vi "Chain of Responsiblility Example.vi"() -> ()   [LabVIEW 2014]
uses:
  user.lib/_NEVSTOP/Communicable State Machine(CSM)/_Support/Typedef/_CSM_MODE.ctl
  user.lib/_NEVSTOP/Communicable State Machine(CSM)/_Support/Priority Queue/Priority Queue.lvclass/Priority Queue.ctl
  user.lib/_NEVSTOP/Communicable State Machine(CSM)/_Support/Typedef/_CSM_GlobalLog_MSG.ctl
  user.lib/_NEVSTOP/Communicable State Machine(CSM)/_Support/Typedef/_CSM_Response Source Message.ctl
  user.lib/_NEVSTOP/Communicable State Machine(CSM)/_Support/Typedef/_CSM_GlobalLog_MSG_TYPE.ctl
  user.lib/_NEVSTOP/Communicable State Machine(CSM)/_Support/CSMQ/_Obtain CSM Data Queue.vi
  user.lib/_NEVSTOP/Communicable State Machine(CSM)/_Support/Priority Queue/Release Priority Queue.vi
  user.lib/_NEVSTOP/Communicable State Machine(CSM)/_Support/Priority Queue/Not a Refnum.vi
  user.lib/_NEVSTOP/Communicable State Machine(CSM)/_Support/Process/CSMP-Async Call.vi
  user.lib/_NEVSTOP/Communicable State Machine(CSM)/_Support/GlobalEvent/GEvt-Generate Status Log.vi
  user.lib/_NEVSTOP/Communicable State Machine(CSM)/_Support/Process/CSMP-Broadcast.vi
  user.lib/_NEVSTOP/Communicable State Machine(CSM)/_Support/GlobalEvent/GEvt-Generate Interrupt Log.vi
  user.lib/_NEVSTOP/Communicable State Machine(CSM)/_Support/GlobalEvent/GEvt-Generate Register Log.vi
  user.lib/_NEVSTOP/Communicable State Machine(CSM)/_Support/Process/CSMP-Register Status.vi
  user.lib/_NEVSTOP/Communicable State Machine(CSM)/_Support/GlobalEvent/GEvt-Generate Unregister Log.vi
  user.lib/_NEVSTOP/Communicable State Machine(CSM)/_Support/Process/CSMP-Unregister Status.vi
  user.lib/_NEVSTOP/Communicable State Machine(CSM)/_Support/Process/CSMP-Sync Call.vi
  user.lib/_NEVSTOP/Communicable State Machine(CSM)/_Support/CSMQ/_CSMObj-Unlock.vi
  user.lib/_NEVSTOP/Communicable State Machine(CSM)/_Support/Process/CSMP-PostPostMsg.vi
  user.lib/_NEVSTOP/Communicable State Machine(CSM)/_Support/Process/CSMP-PostSendMsg.vi
  user.lib/_NEVSTOP/Communicable State Machine(CSM)/_Support/CSMQ/_CSMObj-Lock State.vi
  user.lib/_NEVSTOP/Communicable State Machine(CSM)/_Support/Common/Splite Reason String Part.vi
  user.lib/_NEVSTOP/Communicable State Machine(CSM)/_Support/Common/Trim Single line Text.vi
  user.lib/_NEVSTOP/Communicable State Machine(CSM)/_Support/CSMQ/_CSMOFGV Release.vi
  user.lib/_NEVSTOP/Communicable State Machine(CSM)/_Support/Common/Remove Comments from Line.vi
  user.lib/_NEVSTOP/Communicable State Machine(CSM)/_Support/Common/Splite Single-line Message.vi
  user.lib/_NEVSTOP/Communicable State Machine(CSM)/_Support/Common/Parse Next Single-line State.vi
  user.lib/_NEVSTOP/Communicable State Machine(CSM)/_Support/CSMQ/_CSMObj-Log Error if in a Remote Session.vi
  user.lib/_NEVSTOP/Communicable State Machine(CSM)/_Support/CSMQ/_CSMOFGV Obtain.vi
  user.lib/_NEVSTOP/Communicable State Machine(CSM)/_Support/GlobalEvent/GEvt-Generate State Change Log.vi
  user.lib/_NEVSTOP/Communicable State Machine(CSM)/_Support/GlobalEvent/GEvt-Generate Remaining States Log.vi
  user.lib/_NEVSTOP/Communicable State Machine(CSM)/_Support/GlobalEvent/GEvt-Generate Complete Log.vi
  user.lib/_NEVSTOP/Communicable State Machine(CSM)/AdvanceAPI/CSM - Revert Arguments-Safe String.vi
  user.lib/_NEVSTOP/Communicable State Machine(CSM)/_Support/Priority Queue/Obtain Priority Queue.vi
  user.lib/_NEVSTOP/Communicable State Machine(CSM)/_Support/CSMQ/_CSMObj-Message Check.vi
  user.lib/_NEVSTOP/Communicable State Machine(CSM)/_Support/FGV-BroadcastRegistry/Cache-Broadcast Registry Search Result.vi
  user.lib/_NEVSTOP/Communicable State Machine(CSM)/AdvanceAPI/CSM - Register Status Change.vi
  user.lib/_NEVSTOP/Communicable State Machine(CSM)/AdvanceAPI/CSM - Unregister Status Change.vi
  user.lib/_NEVSTOP/Communicable State Machine(CSM)/Utility/uuid.vi
  user.lib/_NEVSTOP/Communicable State Machine(CSM)/_Support/Common/CSM-Name to CSM-Mode.vi
  user.lib/_NEVSTOP/Communicable State Machine(CSM)/AdvanceAPI/CSM - Keywords.vi
  user.lib/_NEVSTOP/Communicable State Machine(CSM)/_Support/GlobalEvent/FGV-GlobalEventRef.vi
  user.lib/_NEVSTOP/Communicable State Machine(CSM)/_Support/CSMQ/_CSMOFGV.vi
  user.lib/_NEVSTOP/Communicable State Machine(CSM)/_Support/CSMQ/_CSMOFGV Dequeue.vi
  user.lib/_NEVSTOP/Communicable State Machine(CSM)/Utility/Build Error Cluster.vi
  user.lib/_NEVSTOP/Communicable State Machine(CSM)/_Support/CSMQ/_CSMObj-Enqueue Cross-Module Message.vi
  user.lib/_NEVSTOP/Communicable State Machine(CSM)/_Support/GlobalEvent/FGV-StatusChangeEventRef.vi
  user.lib/_NEVSTOP/Communicable State Machine(CSM)/_Support/FGV-BroadcastRegistry/global-Broadcast Cache Change Flag.vi
  user.lib/_NEVSTOP/Communicable State Machine(CSM)/_Support/FGV-BroadcastRegistry/FGV-BroadcastRegistry.vi
  user.lib/_NEVSTOP/Communicable State Machine(CSM)/_Support/Priority Queue/Priority Queue.lvclass
  user.lib/_NEVSTOP/Communicable State Machine(CSM)/Communicable State Machine.lvlib
panel:
  out "Array":T2(array[cluster])
  out "State History 2":string
  out "State History":string
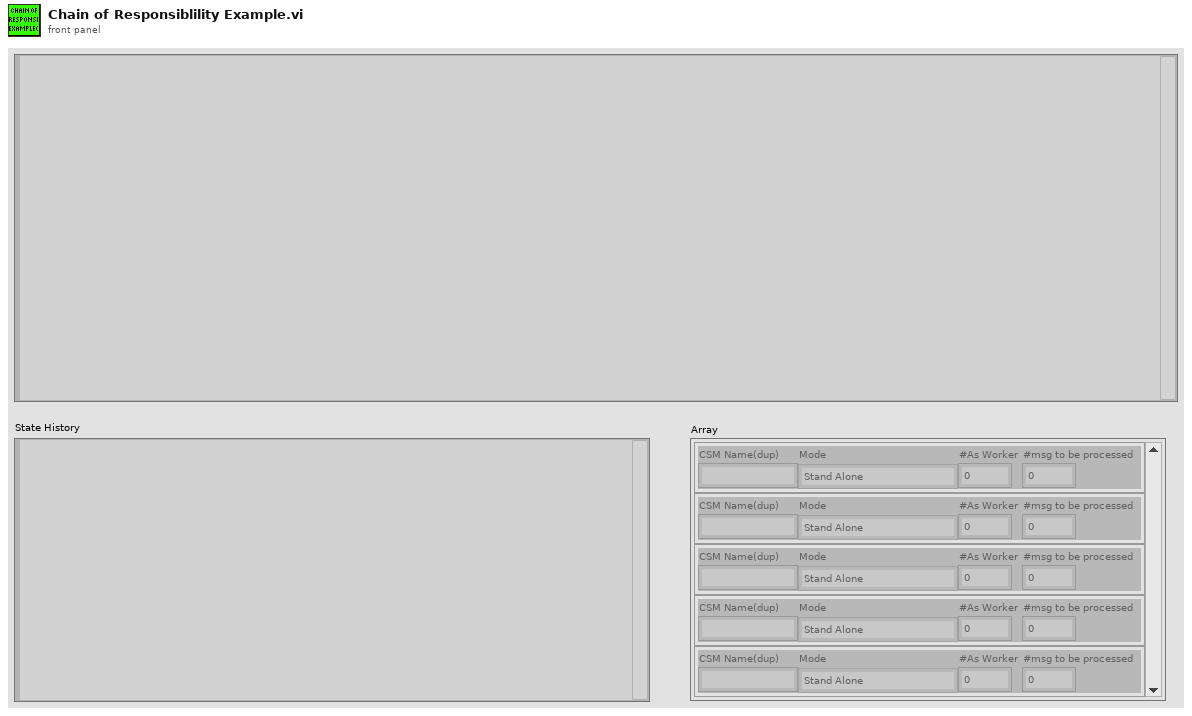
[diagram p1: front panel]
types:
  T1 = typedef "Communicable State Machine.lvlib/_CSM_MODE.ctl" = enum16{"Stand Alone", "CSM", "Action Worker", "Responsibility Chain", "Responsibility Chain Node"}
  T2 = cluster{"CSM Name(dup)":string, "Mode":T1, "#As Worker":i32, "#msg to be processed":i32}[]
  T3 = enum32{"Invalid", "Standard", "Closed", "Hidden", "Minimized", "Maximized"}
  T4 = enum32{"invalid app kind", "Development System", "Run Time System", "Student Edition", "Embedded LabVIEW", "Evaluation", "Custom"}
  T5 = typedef "Communicable State Machine.lvlib/_CSM_Response Source Message.ctl" = cluster{"‘State":string, "’Arguments":string, "’Error":errorcluster}
  T6 = cluster{"Core":cluster{"Current VI Reference":refnum<vi>, "Close Panel on Exit?":bool}, "Your Boolean data":bool, "Your string data":string}
  T7 = cluster{"Current VI Reference":refnum<vi>, "Close Panel on Exit?":bool}
  T8 = typedef "Communicable State Machine.lvlib/_CSM_GlobalLog_MSG.ctl" = cluster{"Name(\"\" to use uuid)":string, "Current State":string, "Arguments":string, "Source Message":T5, "Source Module":string, "Complete(T)/Start(F)":bool, "LogType":T9}
  T9 = typedef "Communicable State Machine.lvlib/_CSM_GlobalLog_MSG_TYPE.ctl" = enum16{"User Log", "State Change", "Status", "Interrupt", "Register", "Unregister"}
  T10 = cluster{"CSM Name(dup)":string, "Mode":T1, "#As Worker":i32, "#msg to be processed":i32}
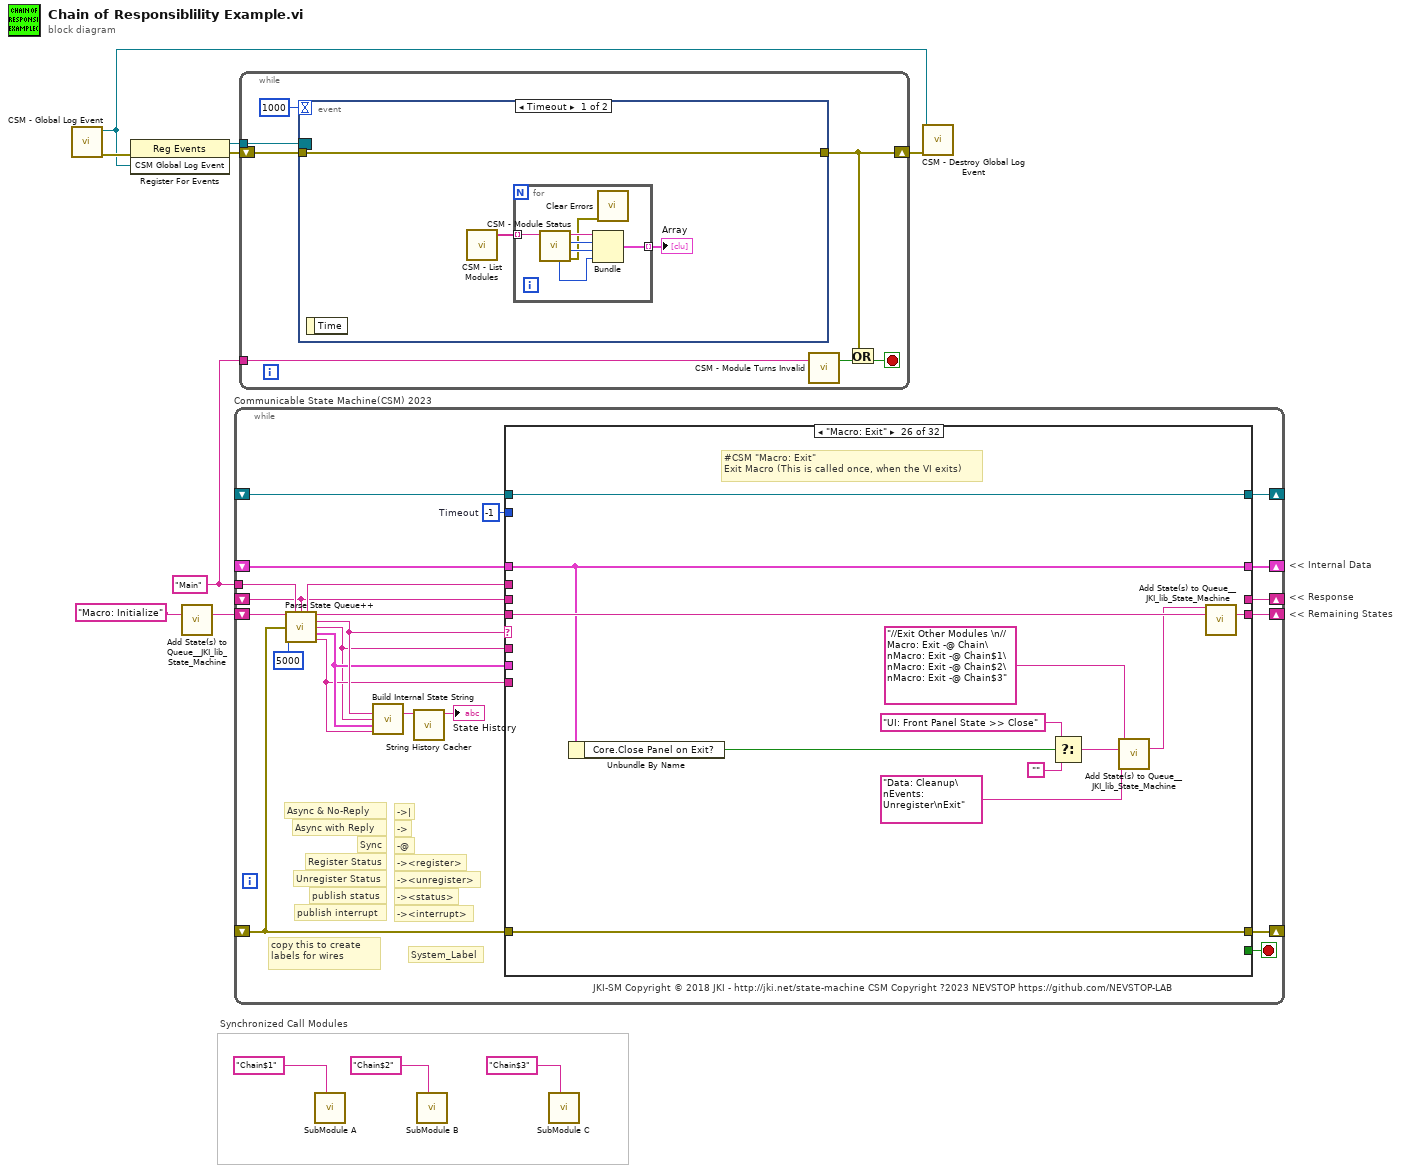
[diagram p0: block diagram]
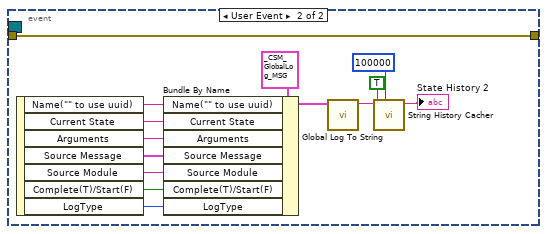
[diagram p2: hidden frame]
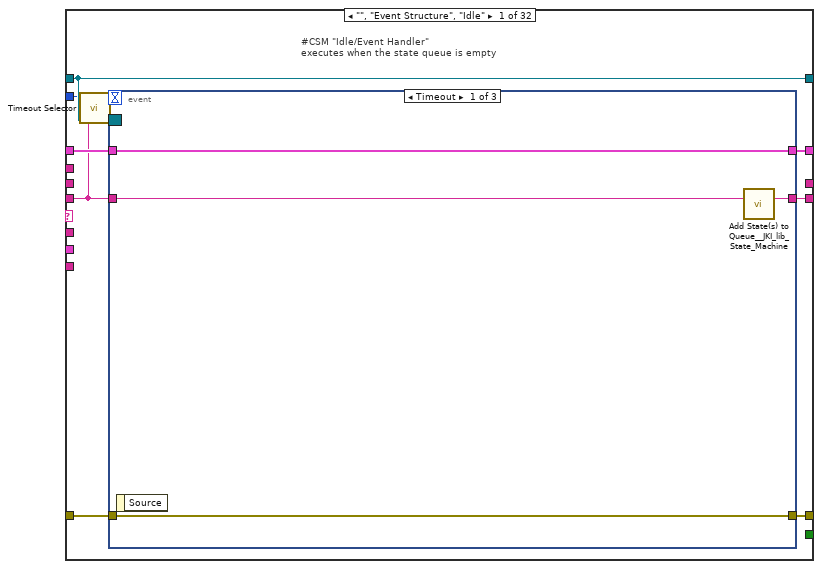
[diagram p3: hidden frame]
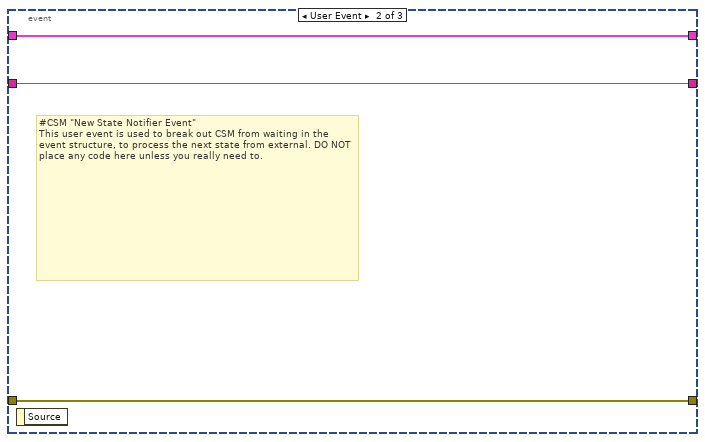
[diagram p4: hidden frame]
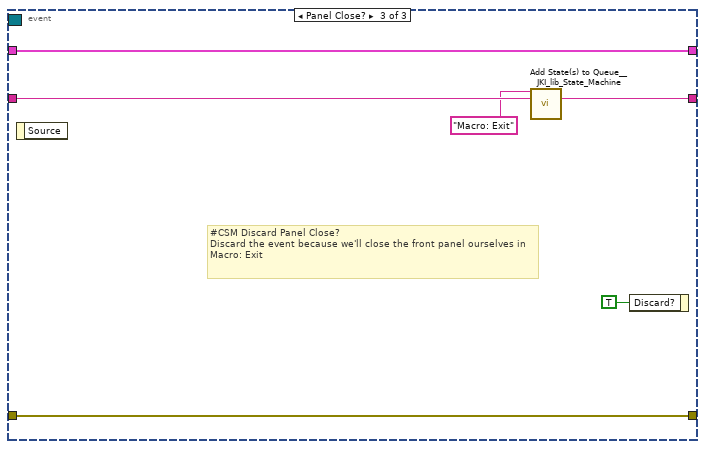
[diagram p5: hidden frame]
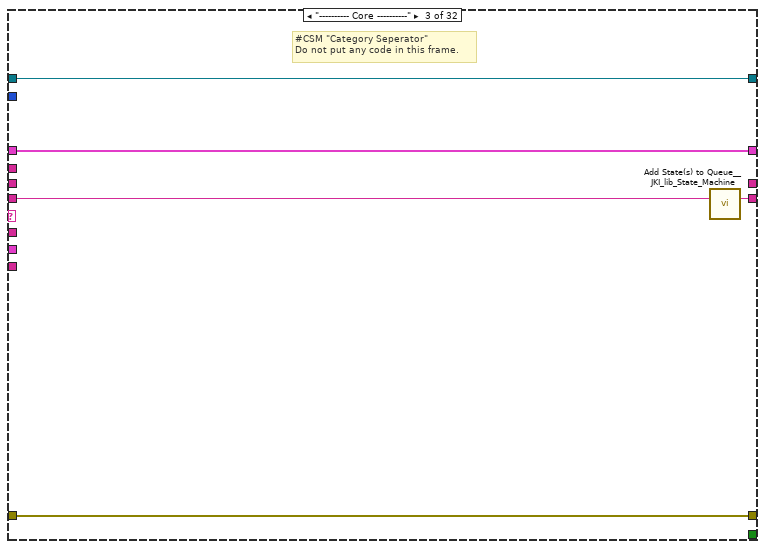
[diagram p7: hidden frame]
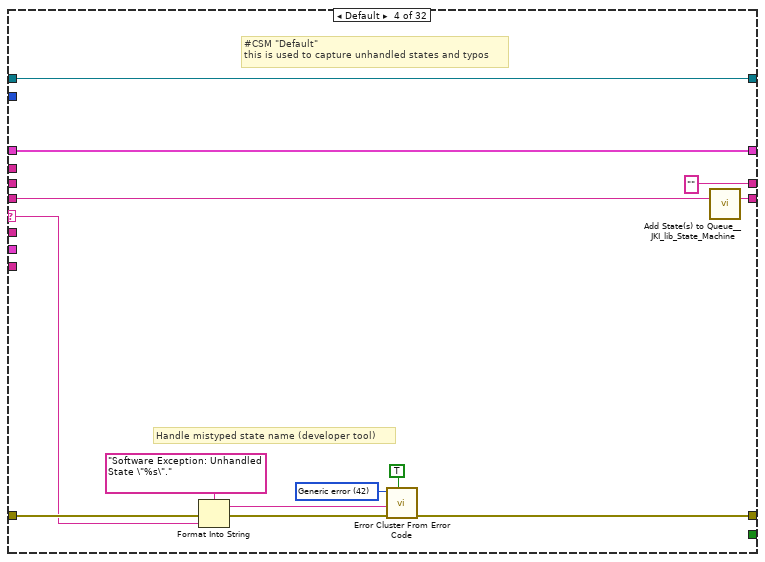
[diagram p8: hidden frame]
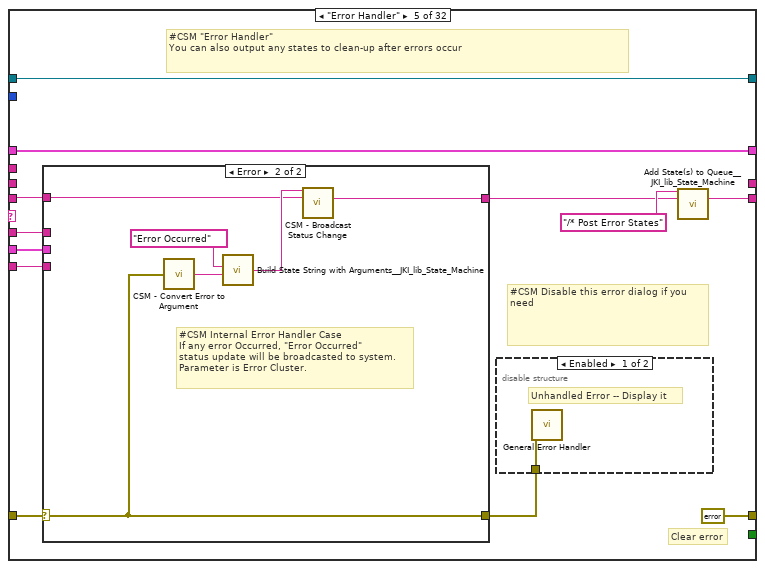
[diagram p9: hidden frame]
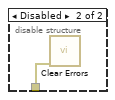
[diagram p10: hidden frame]
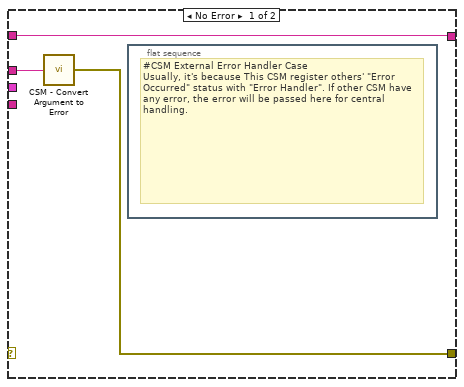
[diagram p11: hidden frame]
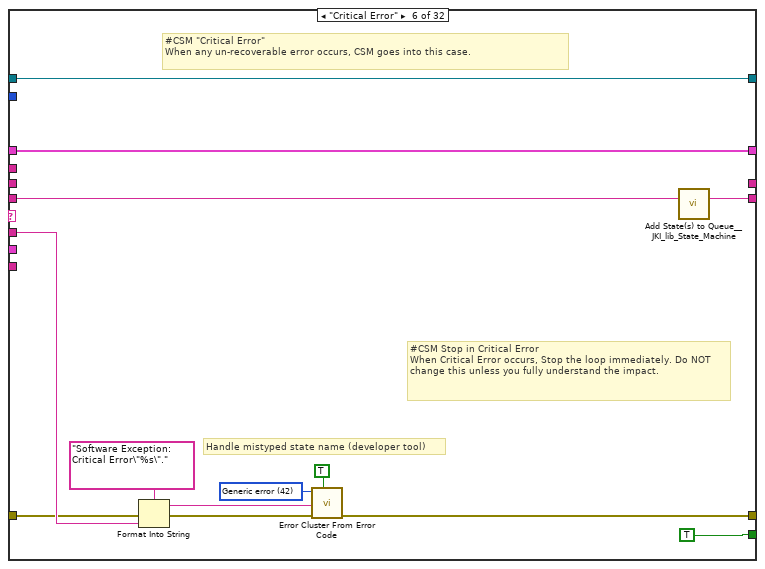
[diagram p12: hidden frame]
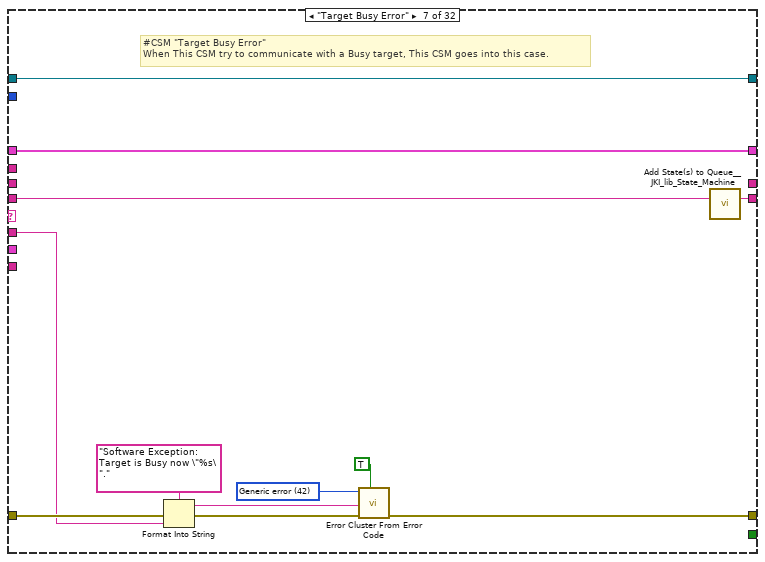
[diagram p13: hidden frame]
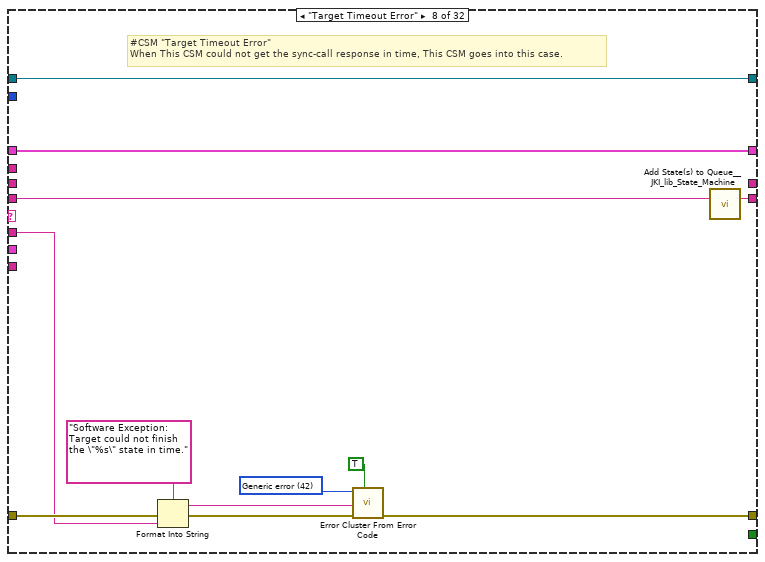
[diagram p14: hidden frame]
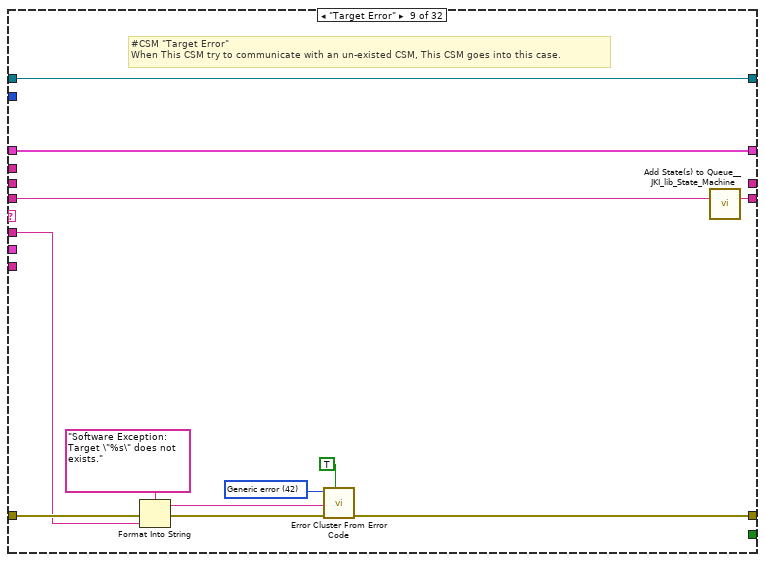
[diagram p15: hidden frame]
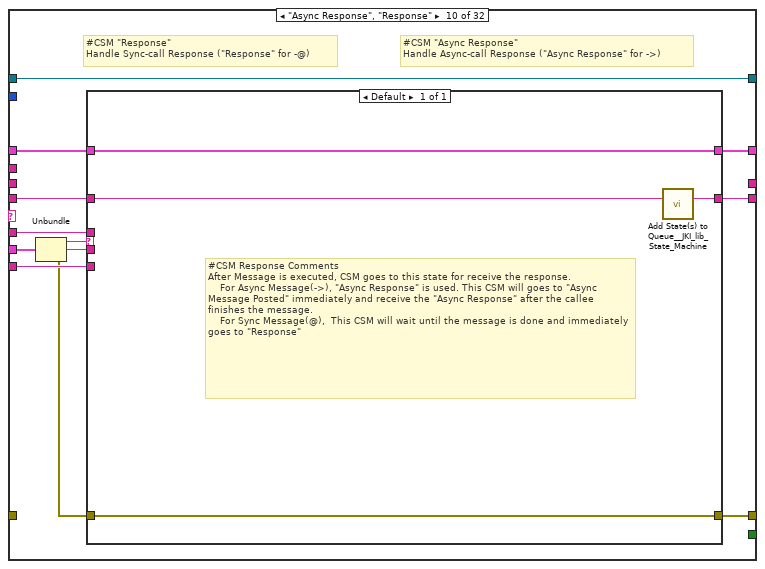
[diagram p16: hidden frame]
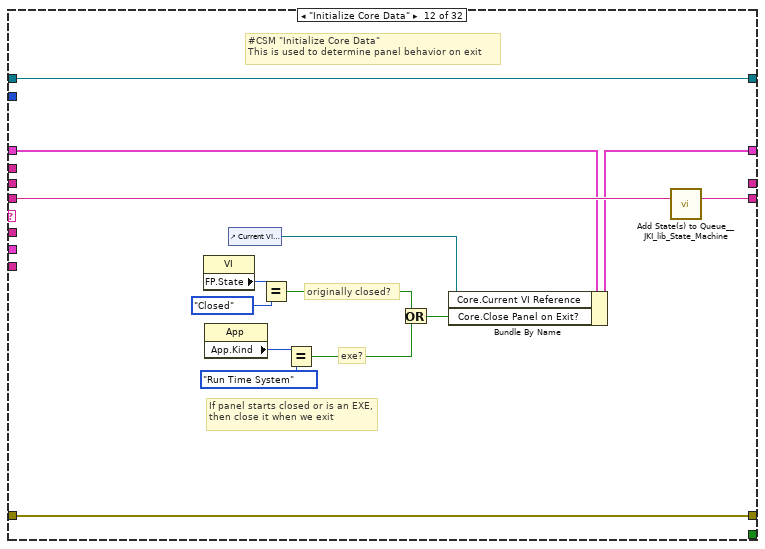
[diagram p18: hidden frame]
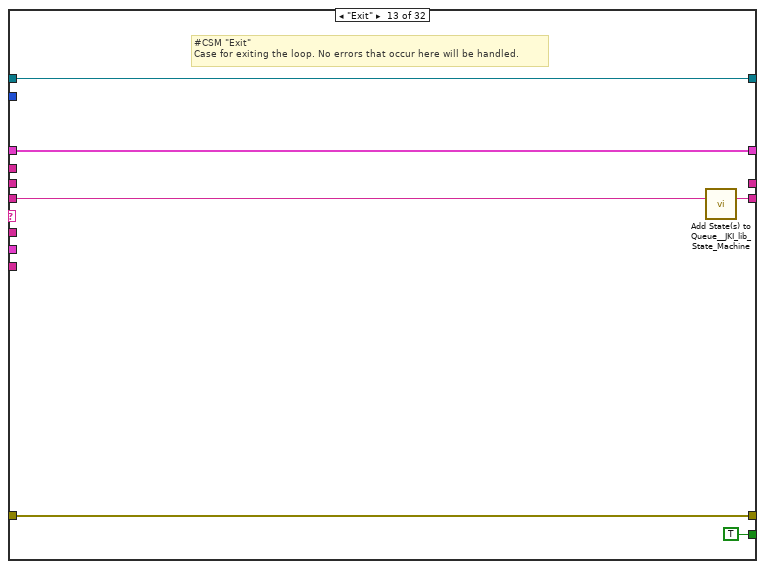
[diagram p19: hidden frame]
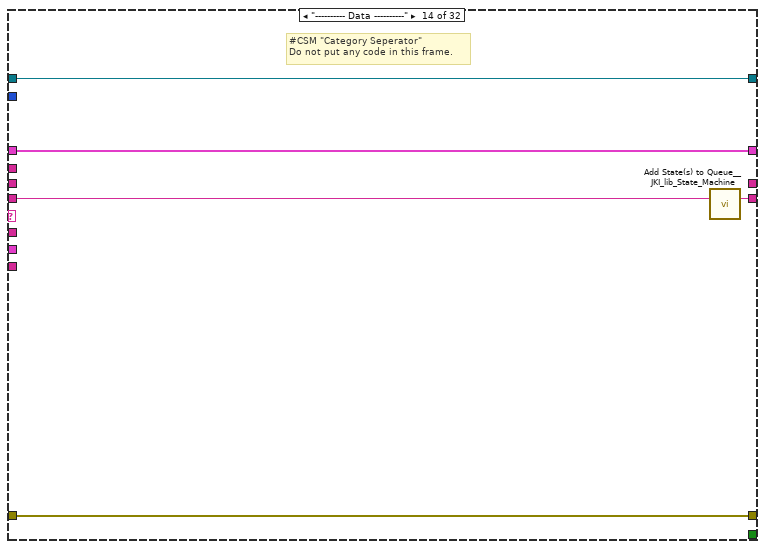
[diagram p20: hidden frame]
diagram:
  w1 = "Main" ("Name(\"\" to use uuid)")
  # "Synchronized Call Modules"
  # "<< Internal Data"
  # "<< Response"
  # "<< Remaining States"
  n1 = call "CSM - Global Log Event.vi"() -> ("Error out"=w3:errorcluster, "CSM Global Log Event"=w2:refnum<user-event>)  [unwired: 10 in]
  n2 = register-events(error in=w3, w2) -> (reference out=w6:refnum<event-registration>, error out=w5:errorcluster)  [unwired: 1 in]
  n3 = call <vilib>:"Add State(s) to Queue__JKI_lib_State_Machine.vi"("State(s) in (\"\")"="Macro: Initialize" ("Init State(\"Macro: Initialize\")")) -> ("States Out"=w11:string)  [unwired: 14 in]
  n4 = while "Communicable State Machine(CSM) 2023" {
    shift-right: [w28] -> _
    shift-left: _ -> [w27]
    shift-right: [w31] -> _
    shift-left: _ -> [w25]
    shift-right: [w30] -> _
    shift-left: w11 -> [w32]
    tunnel: w1 -> [w20]
    shift-right: [w23] -> _
    shift-left: _ -> [w13]
    shift-right: [w22] -> _
    shift-left: _ -> [w21]
    stop <- w29 stop-if-true
    w26 = -1  # Timeout
    # "-><interrupt>"
    # "-><status>"
    # "-><unregister>"
    # "-><register>"
    # "-@"
    # "->"
    # "->|"
    # "publish interrupt"
    # "publish status"
    # "Unregister Status"
    # "Register Status"
    # "Sync"
    # "Async with Reply"
    # "Async & No-Reply"
    # "copy this to create labels for wires"
    # "System_Label"
    # "JKI-SM Copyright © 2018 JKI - http://jki.net/state-machine CSM Copyright ?2023 NEVSTOP https://github.com/NEVSTOP-LAB"
    n5 = call "Parse State Queue++.vi"("State Queue"=w32, "Name(\"\" to use uuid)"=w20, "Response Arguments"=w13, "Error In (no error)"=w25, "Response Timeout(5000ms)"=5000 ("Response Timeout(1000ms)")) -> ("Name Used"=w14:string, "Remaining States"=w33:string, "Current State"=w17:string, "Arguments"=w12:string, ">> Response Source Message >>"=w16:T5, ">> Source CSM >>"=w15:string)  [unwired: 5 in]
    n6 = call "Build Internal State String.vi"("State"=w17, "Arguments (\"\")"=w12, ">> Response Source Message >>"=w16, "Source (\"\")"=w15) -> ("State with Arguments"=w18:string)  [unwired: 11 in]
    n7 = call "String History Cacher.vi"("String"=w18) -> ("String Cache"=→"State History":string)  [unwired: 10 in]
    n8 = case shown="\"Macro: Exit\"" w17 {
      selector: w17 -> [_ _ _ w67 _ _ _ _ _ _ _ _ _ _ _ _ _ _ _ _ _ _ _ _ _ _ _ _ _ _ _ _]
      tunnel: w33 -> [w34 w59 w64 w71 w82 w112 w115 w132 w144 w159 w168 w183 w189 w194 w202 w209 w214 w221 w225 w231 w236 w243 w259 w329 w335 w347 w350 w355 w359 w365 w370 w375]
      tunnel: w12 -> [_ _ _ _ w80 w105 w117 w128 w140 w153 _ _ _ _ _ _ _ _ _ _ _ w238 w253 _ _ _ _ _ _ _ _ _]
      tunnel: w27 -> [w41 w58 w61 w69 w88 w113 w119 w130 w142 w157 w167 w176 w187 w191 _ w204 w211 w220 w224 w228 w234 w241 w255 w326 w332 w344 w349 w354 w358 w362 w367 w372]
      tunnel: [w40 w57 w62 w73 errorcluster {"status"=FALSE, "code"=0, "source"=""} ("error out") w101 w114 w126 w138 w156 w169 w180 w186 w192 w199 w205 w212 w215 w223 w229 w233 w239 w256 w327 w333 w345 w351 w356 w360 w363 w368 w373] -> w31
      tunnel: w25 -> [w39 w57 w62 w72 w86 w102 w121 w133 w145 _ w169 w180 w186 w192 w199 w206 w212 _ w226 w229 w233 w240 w257 w327 w333 w345 w351 w356 w360 w363 w368 w373]
      tunnel: [w42 w59 w63 w70 w84 w111 w120 w131 w143 w160 w168 w182 w188 w193 w201 w208 w213 w221 w225 w230 w235 w242 w258 w328 w334 w346 w350 w355 w359 w364 w369 w374] -> w30
      tunnel: [_ _ _ _ _ TRUE _ _ _ _ _ _ TRUE _ _ _ _ _ _ _ _ _ _ _ _ _ _ _ _ _ _ _] -> w29
      tunnel: [w38 w58 w61 w69 w88 w113 w119 w130 w142 w158 w167 w181 w187 w191 w200 w204 w211 w220 w224 w228 w234 w241 w255 w326 w332 w344 w349 w354 w358 w362 w367 w372] -> w28
      tunnel: w26 -> [w36 _ _ _ _ _ _ _ _ _ _ _ _ _ _ _ _ _ _ _ _ _ _ _ _ _ _ _ _ _ _ _]
      tunnel: w15 -> [_ _ _ _ w79 _ _ _ _ w154 _ _ _ _ _ _ _ _ _ _ _ _ _ _ _ _ _ _ _ _ _ _]
      tunnel: w16 -> [_ _ _ _ w78 _ _ _ _ w155 _ _ _ _ _ _ _ _ _ _ _ _ _ _ _ _ _ _ _ _ _ _]
      tunnel: [_ _ _ "" _ _ _ _ _ _ _ _ _ _ _ _ _ _ _ _ _ _ _ _ _ _ _ "API1 Response" _ _ _ _] -> w23
      tunnel: [w37 w56 w60 w65 w87 w103 w116 w127 w139 w161 w166 w170 w184 w190 w195 w203 w210 w219 w222 w227 w232 w237 w252 w325 w330 w337 w348 w353 w357 w361 w366 w371] -> w22
      tunnel: w21 -> [w37 w56 w60 w65 w87 w103 w116 w127 w139 w161 w166 w170 w184 w190 w195 w203 w210 _ w222 w227 w232 w237 w252 w325 w330 w337 w348 w353 w357 w361 w366 w371]
      tunnel: w14 -> [_ _ _ _ _ _ _ _ _ _ _ _ _ _ _ _ _ w218 _ _ _ _ _ _ _ _ _ _ _ _ _ _]
      tunnel: w13 -> [_ _ _ _ _ _ _ _ _ _ _ _ _ _ _ _ _ _ _ _ _ _ _ _ _ _ _ _ _ _ _ _]
      frame "", "Event Structure", "Idle" {
        # "#CSM \"Idle/Event Handler\"\nexecutes when the state queue is empty"
        n9 = call "Timeout Selector.vi"("Remaining States"=w34, "Timeout Expected"=w36) -> ("Timeout"=w35:i32)  [unwired: 5 in]
        n10 = event shown="[0] Timeout" {
          selector: w37 -> [_ _ _]
          dyn-events: _ -> [_ _ _]
          timeout: w35 -> [_ _ _]
          tunnel: w34 -> [w46 w48 w55]
          tunnel: [w45 w48 w54] -> w42
          tunnel: w41 -> [w43 w49 w52]
          tunnel: [w44 w47 w53] -> w40
          tunnel: w39 -> [w44 w47 w53]
          tunnel: [w43 w49 w52] -> w38
          event Timeout {
            n11 = event-data() -> ()  [unwired: 1 in, 1 out]
            n12 = call <vilib>:"Add State(s) to Queue__JKI_lib_State_Machine.vi"("State(s) in (\"\")"=w46) -> ("States Out"=w45:string)  [unwired: 14 in]
          }
          event User Event {
            # "#CSM \"New State Notifier Event\"\nThis user event is used to break out CSM from waiting in the event structure, to process the next state from external. DO NOT place any code here unless you really need to."
            n13 = event-data() -> ()  [unwired: 1 in, 1 out]
          }
          event Panel Close? {
            # "#CSM Discard Panel Close?\nDiscard the event because we'll close the front panel ourselves in Macro: Exit"
            n14 = event-data() -> ()  [unwired: 1 in, 1 out]
            n15 = call <vilib>:"Add State(s) to Queue__JKI_lib_State_Machine.vi"("State(s) in Front (\"\")"="Macro: Exit", "State(s) in (\"\")"=w55) -> ("States Out"=w54:string)  [unwired: 13 in]
            n16 = event-data("Discard?"=TRUE) -> ()  [unwired: 1 in, 1 out]
          }
        }
      }
      frame "CSM Documentation" {
        # "#CSM \"Documentation\"\nCase for holding CSM Documenation"
        # "CSM Documentation"
        # "#CSM Commenting\nTo add a comment use \"//\" or \"#\" and all text to the right will be ignored\n\nCommenting Example:\nUI: Initialize // This initializes the UI\n// Another comment line"
        # "#CSM State Syntax\n\n    // Local Message Example\n    DoSth: DoA >> Arguments\n\n    // Sync Call Example\n    API: xxxx >> Arguments -@ TargetModule\n\n    // Async Call Example\n    API: xxxx >> Arguments -> TargetModule\n\n    // Async Call without Reply Example\n    API: xxxx >> Arguments ->| TargetModule\n\n    // Broadcast normal status:\n    Status >> StatusArguments  -><status>\n\n    // Broadcast Interrupt status:\n    Interrupt >> StatusArguments  -><interrupt>\n\n    // Register Source Module's status to Handler Module\n    Status@Source Module >> Handler Module@Handler Module -><register>\n\n    // Unegister Source Module's status\n    Status@Source Module >> Handler Module -><unregister>"
        # "#CSM README FIRST\n\nCSM is a LabVIEW application framework that builds upon JKI State Machine (CSM). It follows the pattern of CSM and extends the keywords to describe message communication between CSM modules, including concepts such as Sync-Message, Async-Message, Subscription/Unsubscription of status - essential elements for creating reusable code modules. For more information, please visit the CSM wiki: https://github.com/NEVSTOP-LAB/JKI-State-Machine-Plus-Plus/wiki\n\nFor instructions on JKI State Machine, visit: \n    http://jki.net/state-machine/\nFor information about CSM, visit: \n    https://github.com/NEVSTOP-LAB"
      }
      frame "---------- Core ----------" {
        # "#CSM \"Category Seperator\"\nDo not put any code in this frame."
        n17 = call <vilib>:"Add State(s) to Queue__JKI_lib_State_Machine.vi"("State(s) in (\"\")"=w64) -> ("States Out"=w63:string)  [unwired: 14 in]
      }
      frame Default {
        w76 = 42 items=["No error", "Argument error", "Memory is full", "Out of zone", "End of file", "File already open", "Generic file I/O error", "File not found", "File permission error", "Disk is full", "Duplicate path", "Too many files open", "System feature not enabled", "Resource file not found", "Cannot add resource", "Resource not found", "Image not found", "Image memory error", "Pen does not exist", "Config type invalid", "Config token not found", "Config parse error", "Config memory error", "Bad external code format", "Bad external code offset", "External code not present", "Null window", "Destroy window error", "Null menu", "Print aborted", "Bad print record", "Print driver error", "Windows error during printing", "Memory error during printing", "Print dialog error", "Generic print error", "Invalid device refnum", "Device not found", "Device parameter error", "Device unit error", "Cannot open device", "Device call aborted", "Generic error", "Cancelled by user", "Object ID too low", "Object ID too high", "Object not in heap", "Unknown heap", "Unknown object (invalid DefProc)", "Unknown object (DefProc not in table)", "Message out of range", "Invalid (null) method", "Unknown message", "Manager call not supported", "Bad address", "Network operation in progress", "Network operation timed out", "Connection is busy", "Network attribute not supported", "Network error", "Address in use", "System out of memory", "Connection aborted", "Connection refused", "Not connected", "Already connected", "Connection closed", "Initialization error (interapplication manager)", "Bad occurrence", "Wait on unbound occurrence handler", "Occurrence queue overflow", "Datalog type conflict", "Unused", "Unrecognized type (interapplication manager)", "Memory corrupt", "Failed to make temporary DLL", "Old CIN version", "Drag socket not found", "Failed to load drop-object", "Failed to register OLE object", "Failed to release OLE object", "Format specifier type mismatch", "Unknown format specifier", "Too few format specifiers", "Too many format specifiers", "Scan failed", "Newer CIN version", "Error converting to variant", "Runtime menu error", "Password tampered", "Variant attribute not found", "Incompatible variant data type", "Event data is not available", "Event Store is not present", "Occurrence is not found", "Event Queue is not created", "Event info is not available", "Refnum passed is NULL", "Error retrieving Class GUID", "Error retrieving CoClass GUID", "Error retrieving TypeLib GUID.", "Bad built application magic bytes.", "Specific driver is different from the specific driver associated with the Logical Name.", "There is no session opened to the class driver.", "Max Error", "MAX - Error with config objects", "MAX - Error loading configuration", "MAX - Group not supported"]
        # "#CSM \"Default\"\nthis is used to capture unhandled states and typos"
        # "Handle mistyped state name (developer tool)"
        n18 = Format Into String(format string="Software Exception: Unhandled State \"%s\"." ("message"), error in=w72, w67) -> (resulting string=w75:string, error out=w74:errorcluster)  [unwired: 1 in]
        n19 = call <vilib>:"Error Cluster From Error Code.vi"("show call chain? (False)"=TRUE, "error in (no error)"=w74, "error message (\"\")"=w75, "error code (0)"=w76) -> ("error out"=w73:errorcluster)  [unwired: 5 in]
        n20 = call <vilib>:"Add State(s) to Queue__JKI_lib_State_Machine.vi"("State(s) in (\"\")"=w71) -> ("States Out"=w70:string)  [unwired: 14 in]
      }
      frame "Error Handler" {
        # "#CSM Disable this error dialog if you need"
        # "#CSM \"Error Handler\"\nYou can also output any states to clean-up after errors occur"
        # "Clear error"
        n21 = case shown="Error" w86 {
          selector: w86 -> [_ w95]
          tunnel: [w93 w97] -> w83
          tunnel: w82 -> [w93 w96]
          tunnel: [w92 w95] -> w81
          tunnel: w80 -> [w94 _]
          tunnel: w79 -> [_ _]
          tunnel: w78 -> [_ _]
          frame No Error {
            n22 = call "CSM - Convert Argument to Error.vi"("Argument"=w94) -> ("error"=w92:errorcluster)  [unwired: 4 in]
            n23 = flat-sequence {
              frame #0 {
                # "#CSM External Error Handler Case\nUsually, it's because This CSM register others' \"Error Occurred\" status with \"Error Handler\". If other CSM have any error, the error will be passed here for central handling."
              }
            }
          }
          frame Error {
            # "#CSM Internal Error Handler Case \nIf any error Occurred, \"Error Occurred\" \nstatus update will be broadcasted to system.\nParameter is Error Cluster."
            n24 = call "CSM - Convert Error to Argument.vi"("error in (no error)"=w95) -> ("Arguments"=w99:string)  [unwired: 4 in]
            n25 = call <vilib>:"Build State String with Arguments__JKI_lib_State_Machine.vi"("Arguments (\"\")"=w99, "State"="Error Occurred" ("Status with Arguments")) -> ("State with Arguments"=w98:string)  [unwired: 4 in]
            n26 = call "CSM - Broadcast Status Change.vi"("Status with Arguments"=w98, "State Queue"=w96) -> ("Remaining States"=w97:string)  [unwired: 13 in]
          }
        }
        n27 = disable-structure shown="Enabled" {
          disable-tunnel: w81 -> [w90 w91]
          frame Enabled {
            # "Unhandled Error -- Display it"
            n28 = call <vilib>:"General Error Handler.vi"("error in (no error)"=w90) -> ()  [unwired: 10 in, 5 out]
          }
          frame Disabled {
            n29 = call <vilib>:"Clear Errors.vi"("error in (no error)"=w91) -> ()  [unwired: 6 in, 1 out]
          }
        }
        n30 = call <vilib>:"Add State(s) to Queue__JKI_lib_State_Machine.vi"("State(s) in Front (\"\")"="/* Post Error States", "State(s) in (\"\")"=w83) -> ("States Out"=w84:string)  [unwired: 13 in]
      }
      frame "Critical Error" {
        w109 = 42 items=["No error", "Argument error", "Memory is full", "Out of zone", "End of file", "File already open", "Generic file I/O error", "File not found", "File permission error", "Disk is full", "Duplicate path", "Too many files open", "System feature not enabled", "Resource file not found", "Cannot add resource", "Resource not found", "Image not found", "Image memory error", "Pen does not exist", "Config type invalid", "Config token not found", "Config parse error", "Config memory error", "Bad external code format", "Bad external code offset", "External code not present", "Null window", "Destroy window error", "Null menu", "Print aborted", "Bad print record", "Print driver error", "Windows error during printing", "Memory error during printing", "Print dialog error", "Generic print error", "Invalid device refnum", "Device not found", "Device parameter error", "Device unit error", "Cannot open device", "Device call aborted", "Generic error", "Cancelled by user", "Object ID too low", "Object ID too high", "Object not in heap", "Unknown heap", "Unknown object (invalid DefProc)", "Unknown object (DefProc not in table)", "Message out of range", "Invalid (null) method", "Unknown message", "Manager call not supported", "Bad address", "Network operation in progress", "Network operation timed out", "Connection is busy", "Network attribute not supported", "Network error", "Address in use", "System out of memory", "Connection aborted", "Connection refused", "Not connected", "Already connected", "Connection closed", "Initialization error (interapplication manager)", "Bad occurrence", "Wait on unbound occurrence handler", "Occurrence queue overflow", "Datalog type conflict", "Unused", "Unrecognized type (interapplication manager)", "Memory corrupt", "Failed to make temporary DLL", "Old CIN version", "Drag socket not found", "Failed to load drop-object", "Failed to register OLE object", "Failed to release OLE object", "Format specifier type mismatch", "Unknown format specifier", "Too few format specifiers", "Too many format specifiers", "Scan failed", "Newer CIN version", "Error converting to variant", "Runtime menu error", "Password tampered", "Variant attribute not found", "Incompatible variant data type", "Event data is not available", "Event Store is not present", "Occurrence is not found", "Event Queue is not created", "Event info is not available", "Refnum passed is NULL", "Error retrieving Class GUID", "Error retrieving CoClass GUID", "Error retrieving TypeLib GUID.", "Bad built application magic bytes.", "Specific driver is different from the specific driver associated with the Logical Name.", "There is no session opened to the class driver.", "Max Error", "MAX - Error with config objects", "MAX - Error loading configuration", "MAX - Group not supported"]
        # "#CSM \"Critical Error\"\nWhen any un-recoverable error occurs, CSM goes into this case."
        # "#CSM Stop in Critical Error\nWhen Critical Error occurs, Stop the loop immediately. Do NOT change this unless you fully understand the impact."
        # "Handle mistyped state name (developer tool)"
        n31 = Format Into String(format string="Software Exception: Critical Error\"%s\"." ("message"), error in=w102, w105) -> (resulting string=w108:string, error out=w107:errorcluster)  [unwired: 1 in]
        n32 = call <vilib>:"Error Cluster From Error Code.vi"("show call chain? (False)"=TRUE, "error in (no error)"=w107, "error message (\"\")"=w108, "error code (0)"=w109) -> ("error out"=w101:errorcluster)  [unwired: 5 in]
        n33 = call <vilib>:"Add State(s) to Queue__JKI_lib_State_Machine.vi"("State(s) in (\"\")"=w112) -> ("States Out"=w111:string)  [unwired: 14 in]
      }
      frame "Target Busy Error" {
        w124 = 42 items=["No error", "Argument error", "Memory is full", "Out of zone", "End of file", "File already open", "Generic file I/O error", "File not found", "File permission error", "Disk is full", "Duplicate path", "Too many files open", "System feature not enabled", "Resource file not found", "Cannot add resource", "Resource not found", "Image not found", "Image memory error", "Pen does not exist", "Config type invalid", "Config token not found", "Config parse error", "Config memory error", "Bad external code format", "Bad external code offset", "External code not present", "Null window", "Destroy window error", "Null menu", "Print aborted", "Bad print record", "Print driver error", "Windows error during printing", "Memory error during printing", "Print dialog error", "Generic print error", "Invalid device refnum", "Device not found", "Device parameter error", "Device unit error", "Cannot open device", "Device call aborted", "Generic error", "Cancelled by user", "Object ID too low", "Object ID too high", "Object not in heap", "Unknown heap", "Unknown object (invalid DefProc)", "Unknown object (DefProc not in table)", "Message out of range", "Invalid (null) method", "Unknown message", "Manager call not supported", "Bad address", "Network operation in progress", "Network operation timed out", "Connection is busy", "Network attribute not supported", "Network error", "Address in use", "System out of memory", "Connection aborted", "Connection refused", "Not connected", "Already connected", "Connection closed", "Initialization error (interapplication manager)", "Bad occurrence", "Wait on unbound occurrence handler", "Occurrence queue overflow", "Datalog type conflict", "Unused", "Unrecognized type (interapplication manager)", "Memory corrupt", "Failed to make temporary DLL", "Old CIN version", "Drag socket not found", "Failed to load drop-object", "Failed to register OLE object", "Failed to release OLE object", "Format specifier type mismatch", "Unknown format specifier", "Too few format specifiers", "Too many format specifiers", "Scan failed", "Newer CIN version", "Error converting to variant", "Runtime menu error", "Password tampered", "Variant attribute not found", "Incompatible variant data type", "Event data is not available", "Event Store is not present", "Occurrence is not found", "Event Queue is not created", "Event info is not available", "Refnum passed is NULL", "Error retrieving Class GUID", "Error retrieving CoClass GUID", "Error retrieving TypeLib GUID.", "Bad built application magic bytes.", "Specific driver is different from the specific driver associated with the Logical Name.", "There is no session opened to the class driver.", "Max Error", "MAX - Error with config objects", "MAX - Error loading configuration", "MAX - Group not supported"]
        # "#CSM \"Target Busy Error\"\nWhen This CSM try to communicate with a Busy target, This CSM goes into this case."
        n34 = Format Into String(format string="Software Exception: Target is Busy now \"%s\"." ("message"), error in=w121, w117) -> (resulting string=w123:string, error out=w122:errorcluster)  [unwired: 1 in]
        n35 = call <vilib>:"Error Cluster From Error Code.vi"("show call chain? (False)"=TRUE, "error in (no error)"=w122, "error message (\"\")"=w123, "error code (0)"=w124) -> ("error out"=w114:errorcluster)  [unwired: 5 in]
        n36 = call <vilib>:"Add State(s) to Queue__JKI_lib_State_Machine.vi"("State(s) in (\"\")"=w115) -> ("States Out"=w120:string)  [unwired: 14 in]
      }
      frame "Target Timeout Error" {
        w136 = 42 items=["No error", "Argument error", "Memory is full", "Out of zone", "End of file", "File already open", "Generic file I/O error", "File not found", "File permission error", "Disk is full", "Duplicate path", "Too many files open", "System feature not enabled", "Resource file not found", "Cannot add resource", "Resource not found", "Image not found", "Image memory error", "Pen does not exist", "Config type invalid", "Config token not found", "Config parse error", "Config memory error", "Bad external code format", "Bad external code offset", "External code not present", "Null window", "Destroy window error", "Null menu", "Print aborted", "Bad print record", "Print driver error", "Windows error during printing", "Memory error during printing", "Print dialog error", "Generic print error", "Invalid device refnum", "Device not found", "Device parameter error", "Device unit error", "Cannot open device", "Device call aborted", "Generic error", "Cancelled by user", "Object ID too low", "Object ID too high", "Object not in heap", "Unknown heap", "Unknown object (invalid DefProc)", "Unknown object (DefProc not in table)", "Message out of range", "Invalid (null) method", "Unknown message", "Manager call not supported", "Bad address", "Network operation in progress", "Network operation timed out", "Connection is busy", "Network attribute not supported", "Network error", "Address in use", "System out of memory", "Connection aborted", "Connection refused", "Not connected", "Already connected", "Connection closed", "Initialization error (interapplication manager)", "Bad occurrence", "Wait on unbound occurrence handler", "Occurrence queue overflow", "Datalog type conflict", "Unused", "Unrecognized type (interapplication manager)", "Memory corrupt", "Failed to make temporary DLL", "Old CIN version", "Drag socket not found", "Failed to load drop-object", "Failed to register OLE object", "Failed to release OLE object", "Format specifier type mismatch", "Unknown format specifier", "Too few format specifiers", "Too many format specifiers", "Scan failed", "Newer CIN version", "Error converting to variant", "Runtime menu error", "Password tampered", "Variant attribute not found", "Incompatible variant data type", "Event data is not available", "Event Store is not present", "Occurrence is not found", "Event Queue is not created", "Event info is not available", "Refnum passed is NULL", "Error retrieving Class GUID", "Error retrieving CoClass GUID", "Error retrieving TypeLib GUID.", "Bad built application magic bytes.", "Specific driver is different from the specific driver associated with the Logical Name.", "There is no session opened to the class driver.", "Max Error", "MAX - Error with config objects", "MAX - Error loading configuration", "MAX - Group not supported"]
        # "#CSM \"Target Timeout Error\"\nWhen This CSM could not get the sync-call response in time, This CSM goes into this case."
        n37 = Format Into String(format string="Software Exception: Target could not finish the \"%s\" state in time." ("message"), error in=w133, w128) -> (resulting string=w135:string, error out=w134:errorcluster)  [unwired: 1 in]
        n38 = call <vilib>:"Error Cluster From Error Code.vi"("show call chain? (False)"=TRUE, "error in (no error)"=w134, "error message (\"\")"=w135, "error code (0)"=w136) -> ("error out"=w126:errorcluster)  [unwired: 5 in]
        n39 = call <vilib>:"Add State(s) to Queue__JKI_lib_State_Machine.vi"("State(s) in (\"\")"=w132) -> ("States Out"=w131:string)  [unwired: 14 in]
      }
      frame "Target Error" {
        w148 = 42 items=["No error", "Argument error", "Memory is full", "Out of zone", "End of file", "File already open", "Generic file I/O error", "File not found", "File permission error", "Disk is full", "Duplicate path", "Too many files open", "System feature not enabled", "Resource file not found", "Cannot add resource", "Resource not found", "Image not found", "Image memory error", "Pen does not exist", "Config type invalid", "Config token not found", "Config parse error", "Config memory error", "Bad external code format", "Bad external code offset", "External code not present", "Null window", "Destroy window error", "Null menu", "Print aborted", "Bad print record", "Print driver error", "Windows error during printing", "Memory error during printing", "Print dialog error", "Generic print error", "Invalid device refnum", "Device not found", "Device parameter error", "Device unit error", "Cannot open device", "Device call aborted", "Generic error", "Cancelled by user", "Object ID too low", "Object ID too high", "Object not in heap", "Unknown heap", "Unknown object (invalid DefProc)", "Unknown object (DefProc not in table)", "Message out of range", "Invalid (null) method", "Unknown message", "Manager call not supported", "Bad address", "Network operation in progress", "Network operation timed out", "Connection is busy", "Network attribute not supported", "Network error", "Address in use", "System out of memory", "Connection aborted", "Connection refused", "Not connected", "Already connected", "Connection closed", "Initialization error (interapplication manager)", "Bad occurrence", "Wait on unbound occurrence handler", "Occurrence queue overflow", "Datalog type conflict", "Unused", "Unrecognized type (interapplication manager)", "Memory corrupt", "Failed to make temporary DLL", "Old CIN version", "Drag socket not found", "Failed to load drop-object", "Failed to register OLE object", "Failed to release OLE object", "Format specifier type mismatch", "Unknown format specifier", "Too few format specifiers", "Too many format specifiers", "Scan failed", "Newer CIN version", "Error converting to variant", "Runtime menu error", "Password tampered", "Variant attribute not found", "Incompatible variant data type", "Event data is not available", "Event Store is not present", "Occurrence is not found", "Event Queue is not created", "Event info is not available", "Refnum passed is NULL", "Error retrieving Class GUID", "Error retrieving CoClass GUID", "Error retrieving TypeLib GUID.", "Bad built application magic bytes.", "Specific driver is different from the specific driver associated with the Logical Name.", "There is no session opened to the class driver.", "Max Error", "MAX - Error with config objects", "MAX - Error loading configuration", "MAX - Group not supported"]
        # "#CSM \"Target Error\"\nWhen This CSM try to communicate with an un-existed CSM, This CSM goes into this case."
        n40 = Format Into String(format string="Software Exception: Target \"%s\" does not exists." ("message"), error in=w145, w140) -> (resulting string=w147:string, error out=w146:errorcluster)  [unwired: 1 in]
        n41 = call <vilib>:"Error Cluster From Error Code.vi"("show call chain? (False)"=TRUE, "error in (no error)"=w146, "error message (\"\")"=w147, "error code (0)"=w148) -> ("error out"=w138:errorcluster)  [unwired: 5 in]
        n42 = call <vilib>:"Add State(s) to Queue__JKI_lib_State_Machine.vi"("State(s) in (\"\")"=w144) -> ("States Out"=w143:string)  [unwired: 14 in]
      }
      frame "Async Response", "Response" {
        # "#CSM \"Async Response\"\nHandle Async-call Response (\"Async Response\" for ->)"
        # "#CSM \"Response\"\nHandle Sync-call Response (\"Response\" for -@)"
        n43 = Unbundle(w155) -> ("‘State"=w152:string, "’Arguments"=w151:string, "’Error"=w150:errorcluster)
        n44 = case shown="Default" w152 {
          tunnel: [w162] -> w160
          tunnel: w159 -> [w163]
          tunnel: [w165] -> w158
          tunnel: w157 -> [w165]
          tunnel: [w164] -> w156
          tunnel: w150 -> [w164]
          tunnel: w154 -> [_]
          tunnel: w153 -> [_]
          tunnel: w151 -> [_]
          frame Default {
            # "#CSM Response Comments\nAfter Message is executed, CSM goes to this state for receive the response.\n    For Async Message(->), \"Async Response\" is used. This CSM will goes to \"Async Message Posted\" immediately and receive the \"Async Response\" after the callee finishes the message.\n    For Sync Message(@),  This CSM will wait until the message is done and immediately goes to \"Response\""
            n45 = call <vilib>:"Add State(s) to Queue__JKI_lib_State_Machine.vi"("State(s) in (\"\")"=w163) -> ("States Out"=w162:string)  [unwired: 14 in]
          }
        }
      }
      frame "Async Message Posted" {
        # "#CSM \"Async Message Posted\"\nAfter Async Message is posted (-> or ->| ), CSM goes to this state for post-action.\nYou can use Argument - State to tell which Async Message is called."
      }
      frame "Initialize Core Data" {
        # "#CSM \"Initialize Core Data\"\nThis is used to determine panel behavior on exit"
        # "originally closed?"
        # "exe?"
        # "If panel starts closed or is an EXE, then close it when we exit"
        n46 = property class="VI"() -> ("FP.State"=w173:T3)  [unwired: 2 in, 2 out]
        n47 = property class="App"() -> ("App.Kind"=w179:T4)  [unwired: 2 in, 2 out]
        n48 = control-ref of="Current VI Reference"() -> (w174:refnum<vi>)
        n49 = Equal?(x=w173, y=T3."Closed" ("Front Panel Window:State")) -> (x = y?=w171:bool)
        n50 = Equal?(x=w179, y=T4."Run Time System" ("Application:Kind")) -> (x = y?=w177:bool)
        n51 = Or(x=w171, y=w177) -> (x .or. y?=w175:bool)
        n52 = Bundle By Name(cluster=w176, "Core.Current VI Reference"=w174, "Core.Close Panel on Exit?"=w175) -> (w181:T6)
        n53 = call <vilib>:"Add State(s) to Queue__JKI_lib_State_Machine.vi"("State(s) in (\"\")"=w183) -> ("States Out"=w182:string)  [unwired: 14 in]
      }
      frame "Exit" {
        # "#CSM \"Exit\"\nCase for exiting the loop. No errors that occur here will be handled."
        n54 = call <vilib>:"Add State(s) to Queue__JKI_lib_State_Machine.vi"("State(s) in (\"\")"=w189) -> ("States Out"=w188:string)  [unwired: 14 in]
      }
      frame "---------- Data ----------" {
        # "#CSM \"Category Seperator\"\nDo not put any code in this frame."
        n55 = call <vilib>:"Add State(s) to Queue__JKI_lib_State_Machine.vi"("State(s) in (\"\")"=w194) -> ("States Out"=w193:string)  [unwired: 14 in]
      }
      frame "Data: Initialize" {
        w196 = T7 {"Current VI Reference"=refnum, "Close Panel on Exit?"=FALSE}  # Core
        w198 = TRUE  # Your Boolean data
        w197 = ""  # Your string data
        # "do not delete - used by framework"
        # "Expand Bundle to add new data elements to shift register data."
        # "Add new data here."
        # "Data names and types of shift register data are defined by this bundle."
        # "#CSM \"Data: Initialize\"\nInitialize the shift-register data, here.\n(data names are defined by what you wire into the bundle function)"
        n56 = Bundle("Core"=w196, "Your Boolean data"=w198, "Your string data"=w197) -> (w200:T6)  [unwired: 1 in]
        n57 = call <vilib>:"Add State(s) to Queue__JKI_lib_State_Machine.vi"("State(s) in (\"\")"=w202) -> ("States Out"=w201:string)  [unwired: 14 in]
      }
      frame "Data: Cleanup" {
        # "#CSM \"Data: Cleanup\"\nCleanup any data and references, here.\n(this is called automatically, by the Macro: Exit)"
        n58 = Unbundle By Name(w204) -> ("Core.Current VI Reference"=w207:refnum<vi>)
        n59 = Close Reference(reference=w207, error in (no error)=w206) -> (error out=w205:errorcluster)
        n60 = call <vilib>:"Add State(s) to Queue__JKI_lib_State_Machine.vi"("State(s) in (\"\")"=w209) -> ("States Out"=w208:string)  [unwired: 14 in]
      }
      frame "---------- Events ----------" {
        # "#CSM \"Category Seperator\"\nDo not put any code in this frame."
        n61 = call <vilib>:"Add State(s) to Queue__JKI_lib_State_Machine.vi"("State(s) in (\"\")"=w214) -> ("States Out"=w213:string)  [unwired: 14 in]
      }
      frame "Events: Register" {
        # "#CSM \"Events: Register\"\nRegister user event. New Message Event is registered to break CSM waiting in event structure by default."
        # "#CSM Register New Message Event\nRegister message event to break Waiting in Event structure."
        n62 = call "CSM - Get New State Notifier Event.vi"("Name(\"\" to use uuid) in"=w218) -> ("Error out"=w216:errorcluster, "New State Notifier Event"=w217:refnum<user-event>)  [unwired: 9 in]
        n63 = register-events(error in=w216, w217) -> (reference out=w219:refnum<event-registration>, error out=w215:errorcluster)  [unwired: 1 in]
      }
      frame "Events: Unregister" {
        # "#CSM \"Events: Unregister\"\nUnregister user event."
        n64 = Unregister For Events(event registration refnum=w222, error in=w226) -> (error out=w223:errorcluster)
      }
      frame "---------- UI ----------" {
        # "#CSM \"Category Seperator\"\nDo not put any code in this frame."
        n65 = call <vilib>:"Add State(s) to Queue__JKI_lib_State_Machine.vi"("State(s) in (\"\")"=w231) -> ("States Out"=w230:string)  [unwired: 14 in]
      }
      frame "UI: Initialize" {
        # "#CSM \"UI: Initialize\"\nInitialize the User Interface, here.\n(this is called automatically, by the Macro: Init)"
        n66 = call <vilib>:"Add State(s) to Queue__JKI_lib_State_Machine.vi"("State(s) in (\"\")"=w236) -> ("States Out"=w235:string)  [unwired: 14 in]
      }
      frame "UI: Cursor Set" {
        # "Argument"
        # "#CSM \"UI: Cursor Set\"\nSet and Unset Cursor Busy.\n(Usage: \"UI: Cursor Set >> Busy|Idle\")"
        n67 = disable-structure shown="Default" {
          disable-tunnel: w240 -> [w246 w251]
          disable-tunnel: [w245 w251] -> w239
          disable-tunnel: w238 -> [w244 _]
          frame condition #0 (active) {
            n68 = case shown="\"Busy\"" w244 {
              tunnel: w246 -> [w248 w250]
              tunnel: [w247 w249] -> w245
              frame "Idle", Default {
                n69 = call <vilib>:"Unset Busy.vi"("error in (no error)"=w248) -> ("error out"=w247:errorcluster)  [unwired: 10 in]
              }
              frame "Busy" {
                n70 = call <vilib>:"Set Busy.vi"("error in (no error)"=w250) -> ("error out"=w249:errorcluster)  [unwired: 9 in, 1 out]
              }
            }
          }
          frame condition #1 {
          }
        }
        n71 = call <vilib>:"Add State(s) to Queue__JKI_lib_State_Machine.vi"("State(s) in (\"\")"=w243) -> ("States Out"=w242:string)  [unwired: 14 in]
      }
      frame "UI: Front Panel State" {
        # "Argument"
        # "#CSM \"UI: Front Panel State\"\nSet Front Panel Open or Closed\n(Usage: \"UI: Front Panel State >> Open|Close\")"
        n72 = Unbundle By Name(w255) -> ("Core.Current VI Reference"=w254:refnum<vi>)
        n73 = case shown="\"Minimize\", \"Minimized\"" w253 {
          tunnel: w257 -> [w265 w280 w291 w304 w317]
          tunnel: [w267 w281 w293 w306 w319] -> w256
          tunnel: w254 -> [w266 w278 w292 w305 w318]
          frame "Open", "Standard", Default {
            w260 = T3."Standard" ("State")
            n74 = property class="VI"(reference=w266, error in=w265) -> (reference out=w263:refnum<vi>, error out=w264:errorcluster, "FP.State"=w262:T3)
            n75 = Not Equal?(x=w262, y=w260) -> (x != y?=w261:bool)
            n76 = case shown="True" w261 {
              tunnel: [w271 w273] -> w267
              tunnel: w264 -> [w270 w273]
              tunnel: w263 -> [w269 _]
              tunnel: w260 -> [w268 _]
              frame True {
                n77 = invoke class="VI" method="FP.Open"(reference=w269, error in=w270, "Activate"=TRUE, "State"=w268) -> (error out=w271:errorcluster)  [unwired: 1 in, 4 out]
              }
              frame False {
              }
            }
          }
          frame "Close", "Closed" {
            n78 = property class="VI"(reference=w278, error in=w280) -> (reference out=w277:refnum<vi>, error out=w279:errorcluster, "FP.State"=w275:T3)
            n79 = Not Equal?(x=w275, y=T3."Closed" ("Front Panel Window:State")) -> (x != y?=w274:bool)
            n80 = case shown="True" w274 {
              tunnel: [w282 w285] -> w281
              tunnel: w279 -> [w282 w284]
              tunnel: w277 -> [_ w283]
              frame False {
              }
              frame True {
                n81 = invoke class="VI" method="FP.Close"(reference=w283, error in=w284) -> (error out=w285:errorcluster)  [unwired: 1 in, 2 out]
              }
            }
          }
          frame "Hidden", "Hide" {
            w286 = T3."Hidden" ("State")
            n82 = property class="VI"(reference=w292, error in=w291) -> (reference out=w289:refnum<vi>, error out=w290:errorcluster, "FP.State"=w288:T3)
            n83 = Not Equal?(x=w288, y=w286) -> (x != y?=w287:bool)
            n84 = case shown="True" w287 {
              tunnel: [w297 w298] -> w293
              tunnel: w290 -> [w296 w298]
              tunnel: w289 -> [w295 _]
              tunnel: w286 -> [w294 _]
              frame True {
                n85 = invoke class="VI" method="FP.Open"(reference=w295, error in=w296, "State"=w294) -> (error out=w297:errorcluster)  [unwired: 2 in, 4 out]
              }
              frame False {
              }
            }
          }
          frame "Minimize", "Minimized" {
            w299 = T3."Minimized" ("State")
            n86 = property class="VI"(reference=w305, error in=w304) -> (reference out=w302:refnum<vi>, error out=w303:errorcluster, "FP.State"=w301:T3)
            n87 = Not Equal?(x=w301, y=w299) -> (x != y?=w300:bool)
            n88 = case shown="False" w300 {
              tunnel: [w310 w311] -> w306
              tunnel: w303 -> [w309 w311]
              tunnel: w302 -> [w308 _]
              tunnel: w299 -> [w307 _]
              frame True {
                n89 = invoke class="VI" method="FP.Open"(reference=w308, error in=w309, "State"=w307) -> (error out=w310:errorcluster)  [unwired: 2 in, 4 out]
              }
              frame False {
              }
            }
          }
          frame "Maximize", "Maximized" {
            w312 = T3."Maximized" ("State")
            n90 = property class="VI"(reference=w318, error in=w317) -> (reference out=w315:refnum<vi>, error out=w316:errorcluster, "FP.State"=w314:T3)
            n91 = Not Equal?(x=w314, y=w312) -> (x != y?=w313:bool)
            n92 = case shown="True" w313 {
              tunnel: [w323 w324] -> w319
              tunnel: w316 -> [w322 w324]
              tunnel: w315 -> [w321 _]
              tunnel: w312 -> [w320 _]
              frame True {
                n93 = invoke class="VI" method="FP.Open"(reference=w321, error in=w322, "State"=w320) -> (error out=w323:errorcluster)  [unwired: 2 in, 4 out]
              }
              frame False {
              }
            }
          }
        }
        n94 = call <vilib>:"Add State(s) to Queue__JKI_lib_State_Machine.vi"("State(s) in (\"\")"=w259) -> ("States Out"=w258:string)  [unwired: 14 in]
      }
      frame "---------- Macro ----------" {
        # "#CSM \"Category Seperator\"\nDo not put any code in this frame."
        n95 = call <vilib>:"Add State(s) to Queue__JKI_lib_State_Machine.vi"("State(s) in (\"\")"=w329) -> ("States Out"=w328:string)  [unwired: 14 in]
      }
      frame "Macro: Initialize" {
        w331 = "Data: Initialize\nInitialize Core Data\nEvents: Register\nUI: Initialize\nUI: Front Panel State >> Open"  # Data: Initialize Initialize Core Data Events: Register UI: Initialize UI: Front Panel State >> Open
        # "#CSM \"Macro: Initialize\"\nInitialization Macro (This is called once, when the VI starts)"
        n96 = call <vilib>:"Add State(s) to Queue__JKI_lib_State_Machine.vi"("State(s) in Front (\"\")"=w331, "State(s) in (\"\")"=w335) -> ("States Out"=w334:string)  [unwired: 13 in]
      }
      frame "Macro: Exit" {
        # "#CSM \"Macro: Exit\"\nExit Macro (This is called once, when the VI exits)"
        n97 = Unbundle By Name(w344) -> ("Core.Close Panel on Exit?"=w343:bool)
        n98 = Select(t="UI: Front Panel State >> Close", s=w343, f="") -> (s? t:f=w340:string)
        n99 = call <vilib>:"Add State(s) to Queue__JKI_lib_State_Machine.vi"("State(s) in Front (\"\")"="//Exit Other Modules \n//Macro: Exit -@ Chain\nMacro: Exit -@ Chain$1\nMacro: Exit -@ Chain$2\nMacro: Exit -@ Chain$3", "State(s) in (\"\")"=w340, "State(s) at Back (\"\")"="Data: Cleanup\nEvents: Unregister\nExit") -> ("States Out"=w338:string)  [unwired: 12 in]
        n100 = call <vilib>:"Add State(s) to Queue__JKI_lib_State_Machine.vi"("State(s) in Front (\"\")"=w338, "State(s) in (\"\")"=w347) -> ("States Out"=w346:string)  [unwired: 13 in]
      }
      frame "---------- API ----------" {
        # "#CSM \"Category Seperator\"\nDo not put any code in this frame."
      }
      frame "API: API1" {
        # "#CSM >> Source CSM >>\nIf you need to tell who triggered this state , use this string. If it's this case itself, this string is \"\"."
        # "#CSM >> Arguments >>\nDeal with the parameter if any"
        # "#CSM Response\nConnect this to return the response of your API"
        # "#CSM API Example\nCopy/Rename this case for your own API"
      }
      frame "API: API2" {
        # "#CSM API Example\nCopy/Rename this case for your own API"
      }
      frame "---------- DoSth ----------" {
        # "#CSM \"Category Seperator\"\nDo not put any code in this frame."
        n101 = call <vilib>:"Add State(s) to Queue__JKI_lib_State_Machine.vi"("State(s) in (\"\")"=w365) -> ("States Out"=w364:string)  [unwired: 14 in]
      }
      frame "DoSth: DoA" {
        # "#CSM \"Internal State\"\nThis category is used for holding internal states"
        n102 = call <vilib>:"Add State(s) to Queue__JKI_lib_State_Machine.vi"("State(s) in (\"\")"=w370) -> ("States Out"=w369:string)  [unwired: 14 in]
      }
      frame "DoSth: DoB" {
        # "#CSM \"Internal State\"\nThis category is used for holding internal states"
        n103 = call <vilib>:"Add State(s) to Queue__JKI_lib_State_Machine.vi"("State(s) in (\"\")"=w375) -> ("States Out"=w374:string)  [unwired: 14 in]
      }
    }
  }
  n104 = while {
    tunnel: w6 -> [w382]
    shift-right: [w379] -> w4
    shift-left: w5 -> [w381]
    tunnel: w1 -> [w377]
    stop <- w380 stop-if-true
    n105 = event shown="[0] Timeout" {
      selector: w382 -> [_ _]
      dyn-events: _ -> [_ _]
      timeout: 1000 -> [_ _]
      tunnel: w381 -> [w385 w406]
      tunnel: [w385 w406] -> w379
      event Timeout {
        n106 = event-data() -> ()  [unwired: 1 in, 1 out]
        n107 = call "CSM - List Modules.vi"() -> ("Module Names"=w384:string[])  [unwired: 10 in, 1 out]
        n108 = for {
          tunnel: w384 -> [w392] mode=indexing
          tunnel: [w387] -> w383 mode=indexing
          n109 = call "CSM - Module Status.vi"("CSM Name"=w392) -> ("Error out"=w386:errorcluster, "#As Worker"=w389:i32, "Mode"=w390:T1, "CSM Name(dup)"=w391:string, "#msg to be processed"=w388:i32)  [unwired: 6 in]
          n110 = Bundle("CSM Name(dup)"=w391, "Mode"=w390, "#As Worker"=w389, "#msg to be processed"=w388) -> (w387:T10)  [unwired: 1 in]
          n111 = call <vilib>:"Clear Errors.vi"("error in (no error)"=w386) -> ()  [unwired: 6 in, 1 out]
        }
        "Array" <- w383
      }
      event User Event {
        n112 = event-data() -> ("Name(\"\" to use uuid)"=w401:string, "Current State"=w400:string, "Arguments"=w399:string, "Source Message"=w398:T5, "Source Module"=w397:string, "Complete(T)/Start(F)"=w396:bool, "LogType"=w395:T9)  [unwired: 1 in]
        n113 = Bundle By Name(cluster=T8 {"Name(\"\" to use uuid)"="", "Current State"="", "Arguments"="", "Source Message"={"‘State"="", "’Arguments"="", "’Error"={"status"=FALSE, "code"=0, "source"=""}}, "Source Module"="", "Complete(T)/Start(F)"=FALSE, "LogType"=enum."State Change"} ("Cross CSM Data"), "Name(\"\" to use uuid)"=w401, "Current State"=w400, "Arguments"=w399, "Source Message"=w398, "Source Module"=w397, "Complete(T)/Start(F)"=w396, "LogType"=w395) -> (w393:T8)
        n114 = call "Global Log To String.vi"("Log"=w393) -> ("String"=w402:string)  [unwired: 9 in]
        n115 = call "String History Cacher.vi"("length"=100000, "Include Timestamp(T)"=TRUE ("Include Timestamp(F)"), "String"=w402) -> ("String Cache"=→"State History 2":string)  [unwired: 8 in]
      }
    }
    n116 = call "CSM - Module Turns Invalid.vi"("CSM Name"=w377) -> ("Turn Invalid(Exit)?"=w376:bool)  [unwired: 2 in]
    n117 = Or(x=w379, y=w376) -> (x .or. y?=w380:bool)
  }
  n118 = call "SubModule A.vi"("Name(\"\" to use uuid)"="Chain$1" ("Name(\"\" to use uuid)")) -> ()  [unwired: 11 in]
  n119 = call "SubModule B.vi"("Name(\"\" to use uuid)"="Chain$2" ("Name(\"\" to use uuid)")) -> ()  [unwired: 11 in]
  n120 = call "SubModule C.vi"("Name(\"\" to use uuid)"="Chain$3" ("Name(\"\" to use uuid)")) -> ()  [unwired: 11 in]
  n121 = call "CSM - Destroy Global Log Event.vi"("Error in"=w4, "CSM Global Log Event"=w2) -> ()  [unwired: 9 in, 1 out]
